vi "Create Constant.vi"(0 "Diagram in":refnum<vi>, 2 "location (0, 0)":T1, 5 "Type":variant, 7 "Value":variant, 11 "error in (no error)":errorcluster) -> (4 "Diagram out":refnum<vi>, 6 "Terminal":refnum<vi>, 15 "error out":errorcluster)   [LabVIEW 2015, in "Scripting.lvlib"]
doc: "Creates a Constant at <B>location</B> on <B>Diagram in</B>.\n\n<B>Type</B> is the data type of the created constant and, if <B>Value</B> is unwired, the value as well.\n\n<B>Value</B> is optionally the value of the created constant. This input can be useful if the desired type is easy to obtain (i.e. a typedef), but a specific value of that type is not. Value does not have to be the same type as <B>Type</B>, but must be compatible."
uses:
  Scripting.lvlib
  <vilib>/Utility/miscctls.llb/LVPointTypeDef.ctl
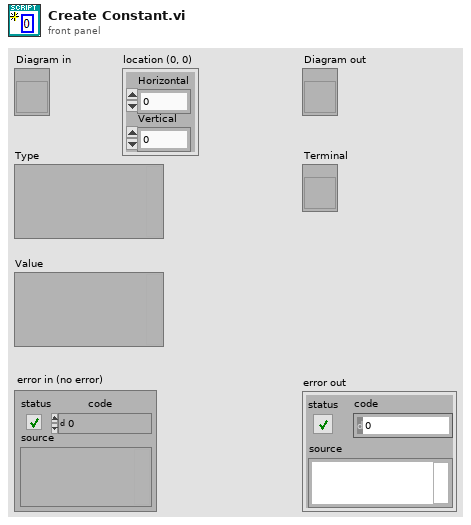
[diagram p1: front panel]
types:
  T1 = typedef "LVPointTypeDef.ctl" = cluster{"Horizontal":i16, "Vertical":i16}
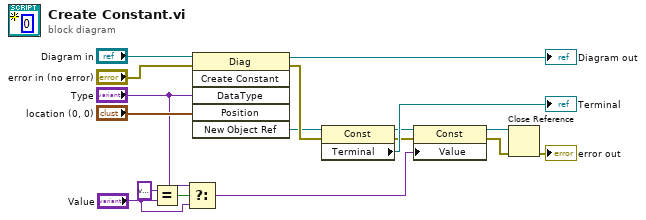
[diagram p0: block diagram]
diagram:
  n1 = Equal?(x=variant, y="Value") -> (x = y?=w9:bool)
  n2 = Select(t="Type", s=w9, f="Value") -> (s? t:f=w6:variant)
  n3 = invoke class="Diag" method="Create Constant"(reference="Diagram in", error in="error in (no error)", "DataType"="Type", "Position"="location (0, 0)") -> (reference out=→"Diagram out":refnum<vi>, error out=w4:errorcluster, "New Object Ref"=w2:refnum<vi>)  [unwired: 2 in, 3 out]
  n4 = property class="Const"(reference=w2, error in=w4) -> (reference out=w1:refnum<vi>, error out=w3:errorcluster, "Terminal"=→"Terminal":refnum<vi>)
  n5 = property class="Const"(reference=w1, error in=w3, "Value"=w6) -> (reference out=w11:refnum<vi>, error out=w13:errorcluster)
  n6 = Close Reference(reference=w11, error in (no error)=w13) -> (error out=→"error out":errorcluster)
